vi "仪器控制.vi"() -> ()   [LabVIEW 2012]
uses:
  <vilib>/Instr/_visa.llb/VISA Configure Serial Port (Instr).vi
panel:
  in  "总持续时间3":dbl
  in  "总持续时间2":dbl
  in  "总持续时间1(s)":dbl=10.0
  in  "Time Resolution(s)":dbl=0.05
  in  "IR":dbl=1.0
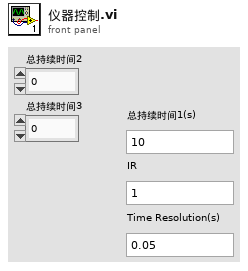
[diagram p1: front panel]
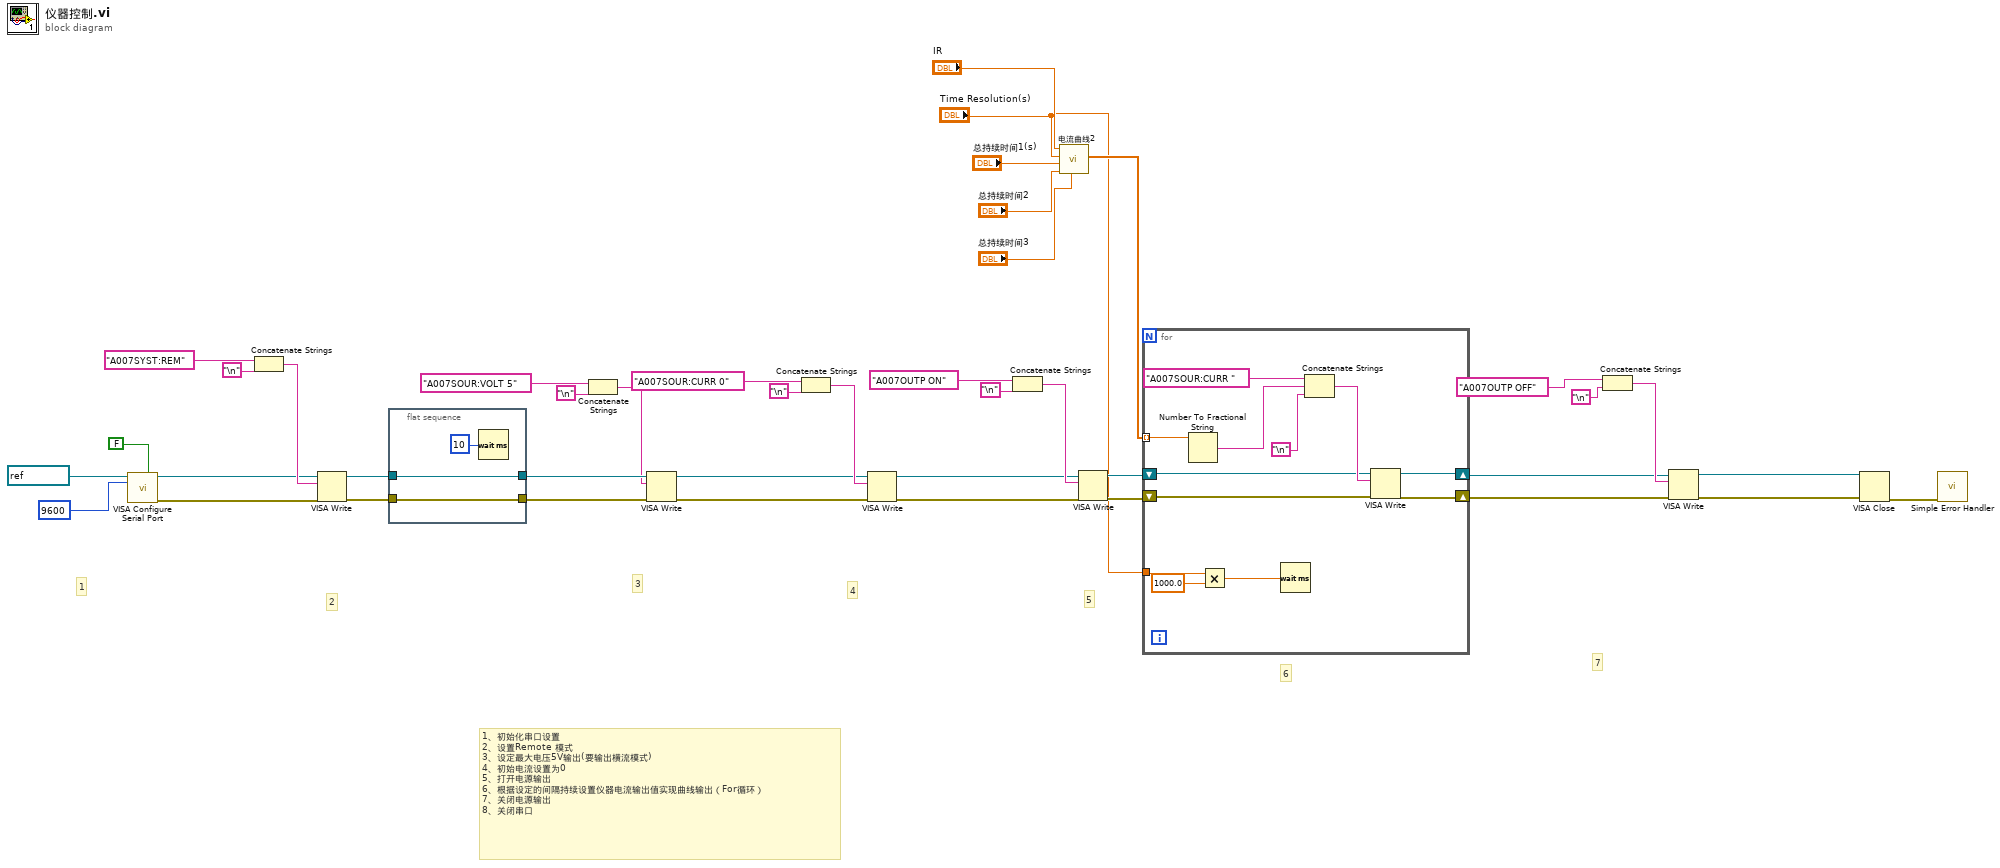
[diagram p0: block diagram]
diagram:
  # "7"
  # "5"
  # "6"
  # "4"
  # "3"
  # "2"
  # "1"
  # "1、初始化串口设置\n2、设置Remote 模式\n3、设定最大电压5V输出(要输出横流模式)\n4、初始电流设置为0\n5、打开电源输出\n6、根据设定的间隔持续设置仪器电流输出值实现曲线输出（For循环）\n7、关闭电源输出\n8、关闭串口"
  n1 = call-poly "VISA Configure Serial Port"("VISA resource name"=refnum<visa-resource-name> "COM3", "Enable Termination\nChar (T)"=FALSE ("Enable Termination\nChar (T)"), "baud rate (9600)"=u32 9600) -> ("VISA resource name out"=w33:refnum<visa-resource-name>, "error out"=w32:errorcluster)  [unwired: 11 in]
  n2 = Concatenate Strings("A007SYST:REM" ("字符串"), "\n") -> (w38:string)
  n3 = VISA Write(VISA resource name=w33, write buffer=w38, error in (no error)=w32) -> (VISA resource name out=w41:refnum<visa-resource-name>, error out=w40:errorcluster)  [unwired: 1 out]
  n4 = flat-sequence {
    tunnel: w41 -> [w43]
    tunnel: [w43] -> w30
    tunnel: w40 -> [w42]
    tunnel: [w42] -> w29
    frame #0 {
      n5 = Wait (ms)(milliseconds to wait=u32 10 ("等待时间（毫秒）")) -> ()  [unwired: 1 out]
    }
  }
  n6 = Concatenate Strings("A007SOUR:VOLT 5" ("字符串"), "\n") -> (w26:string)
  n7 = VISA Write(VISA resource name=w30, write buffer=w26, error in (no error)=w29) -> (VISA resource name out=w22:refnum<visa-resource-name>, error out=w21:errorcluster)  [unwired: 1 out]
  n8 = Concatenate Strings("A007SOUR:CURR 0" ("字符串"), "\n") -> (w25:string)
  n9 = VISA Write(VISA resource name=w22, write buffer=w25, error in (no error)=w21) -> (VISA resource name out=w17:refnum<visa-resource-name>, error out=w16:errorcluster)  [unwired: 1 out]
  n10 = Concatenate Strings("A007OUTP ON" ("字符串"), "\n") -> (w18:string)
  n11 = call "电流曲线2.vi"("总持续时间3"="总持续时间3", "总持续时间2"="总持续时间2", "总持续时间1"="总持续时间1(s)", "时间分辨率"="Time Resolution(s)", "IR"="IR") -> ("最终电流值"=w6:dbl[])  [unwired: 6 in]
  n12 = VISA Write(VISA resource name=w17, write buffer=w18, error in (no error)=w16) -> (VISA resource name out=w15:refnum<visa-resource-name>, error out=w14:errorcluster)  [unwired: 1 out]
  n13 = for {
    tunnel: w6 -> [w51] mode=indexing
    tunnel: "Time Resolution(s)" -> [w49]
    shift-right: [w46] -> w9
    shift-left: w14 -> [w53]
    shift-right: [w45] -> w10
    shift-left: w15 -> [w54]
    n14 = Number To Fractional String(number=w51) -> (F-format string=w50:string)  [unwired: 3 in]
    n15 = Multiply(x=w49, y=1000.0) -> (x*y=w47:dbl)
    n16 = Wait (ms)(milliseconds to wait=w47) -> ()  [unwired: 1 out]
    n17 = Concatenate Strings("A007SOUR:CURR " ("字符串"), w50, "\n") -> (w55:string)
    n18 = VISA Write(VISA resource name=w54, write buffer=w55, error in (no error)=w53) -> (VISA resource name out=w45:refnum<visa-resource-name>, error out=w46:errorcluster)  [unwired: 1 out]
  }
  n19 = Concatenate Strings("A007OUTP OFF" ("字符串"), "\n") -> (w13:string)
  n20 = VISA Write(VISA resource name=w10, write buffer=w13, error in (no error)=w9) -> (VISA resource name out=w8:refnum<visa-resource-name>, error out=w7:errorcluster)  [unwired: 1 out]
  n21 = VISA Close(VISA resource name=w8, error in (no error)=w7) -> (error out=w36:errorcluster)
  n22 = call <vilib>:"Simple Error Handler.vi"("error in (no error)"=w36) -> ()  [unwired: 4 in, 5 out]
